vi "根据监测浓度升序排列.vi"(11 "标液浓度输入":dbl[][](array[numeric])) -> (3 "输出数组":dbl[][](array[numeric]))   [LabVIEW 2016]
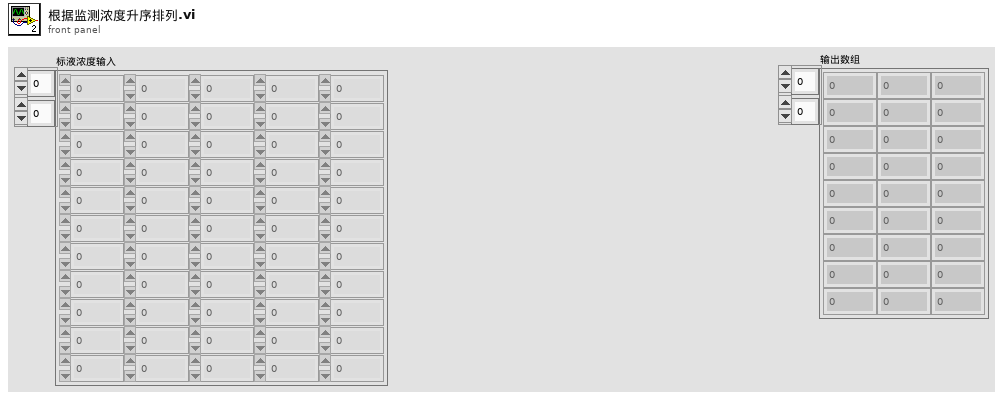
[diagram p1: front panel]
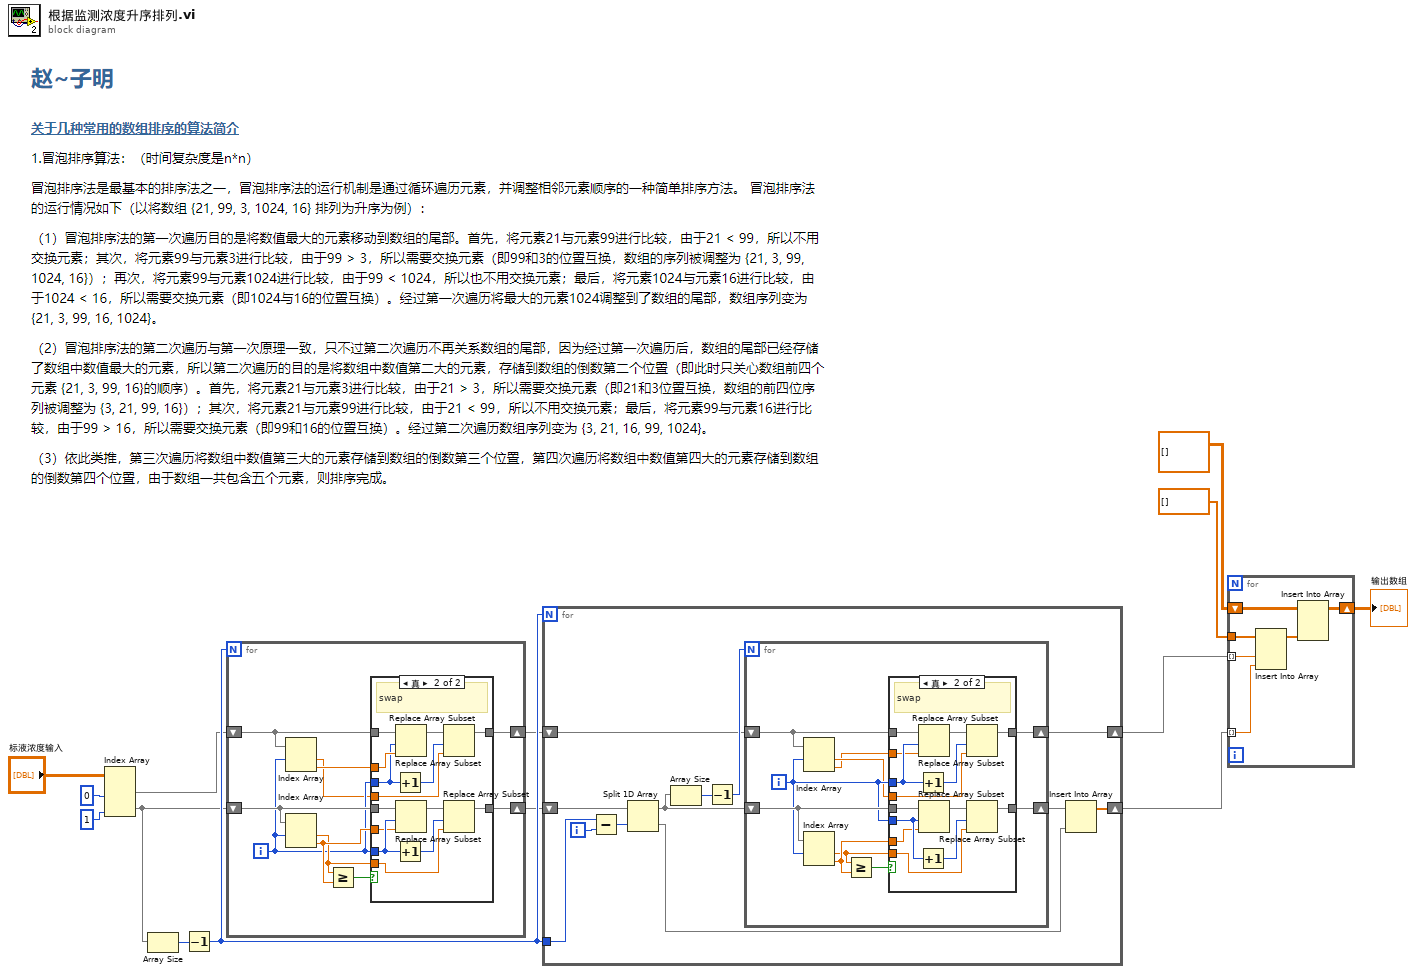
[diagram p0: block diagram]
diagram:
  n1 = Index Array(array="标液浓度输入", index (col) #1=0 ("禁用的索引 (列)"), index (col) #2=1 ("索引 (列)")) -> (element #1=w7:dbl[], element #2=w8:dbl[])  [unwired: 2 in]
  n2 = Array Size(array=w8) -> (size(s)=w11:i32)
  n3 = Decrement(x=w11) -> (x-1=w10:i32)
  n4 = for {
    N: w10 -> [_]
    shift-right: [w21] -> w9
    shift-left: w8 -> [w20]
    shift-right: [w17] -> w6
    shift-left: w7 -> [w19]
    i -> [w16]
    n5 = Index Array(array=w19, index #1=w16) -> (element #1=w15:dbl, element #2=w18:dbl)  [unwired: 1 in]
    n6 = Index Array(array=w20, index #1=w16) -> (element #1=w22:dbl, element #2=w23:dbl)  [unwired: 1 in]
    n7 = Greater Or Equal?(x=w22, y=w23) -> (x >= y?=w24:bool)
    n8 = case shown="真" w24 {
      tunnel: w20 -> [w26 w40]
      tunnel: w16 -> [_ w39]
      tunnel: w23 -> [_ w37]
      tunnel: w22 -> [_ w36]
      tunnel: [w26 w34] -> w21
      tunnel: w19 -> [w25 w30]
      tunnel: [w25 w33] -> w17
      tunnel: w18 -> [_ w29]
      tunnel: w16 -> [_ w28]
      tunnel: w15 -> [_ w27]
      frame False {
      }
      frame True {
        # "swap"
        n9 = Increment(x=w28) -> (x+1=w31:i32)
        n10 = Increment(x=w39) -> (x+1=w38:i32)
        n11 = Replace Array Subset(array=w30, new element=w29, index=w28) -> (w32:dbl[])
        n12 = Replace Array Subset(array=w40, new element=w37, index=w39) -> (w35:dbl[])
        n13 = Replace Array Subset(array=w32, new element=w27, index=w31) -> (w33:dbl[])
        n14 = Replace Array Subset(array=w35, new element=w36, index=w38) -> (w34:dbl[])
      }
    }
  }
  n15 = for {
    N: w10 -> [_]
    shift-right: [w45] -> w1
    shift-left: w9 -> [w50]
    tunnel: w10 -> [w48]
    shift-right: [w41] -> w2
    shift-left: w6 -> [w42]
    i -> [w44]
    n16 = Subtract(x=w48, y=w44) -> (x-y=w43:i32)
    n17 = Split 1D Array(array=w50, index=w43) -> (first subarray=w49:dbl[], second subarray=w46:dbl[])
    n18 = Array Size(array=w49) -> (size(s)=w52:i32)
    n19 = Decrement(x=w52) -> (x-1=w51:i32)
    n20 = for {
      N: w51 -> [_]
      shift-right: [w59] -> w47
      shift-left: w49 -> [w58]
      shift-right: [w57] -> w41
      shift-left: w42 -> [w55]
      i -> [w56]
      n21 = Index Array(array=w55, index #1=w56) -> (element #1=w54:dbl, element #2=w53:dbl)  [unwired: 1 in]
      n22 = Index Array(array=w58, index #1=w56) -> (element #1=w60:dbl, element #2=w61:dbl)  [unwired: 1 in]
      n23 = Greater Or Equal?(x=w60, y=w61) -> (x >= y?=w62:bool)
      n24 = case shown="真" w62 {
        tunnel: w58 -> [w64 w78]
        tunnel: w56 -> [_ w77]
        tunnel: w61 -> [_ w75]
        tunnel: w60 -> [_ w74]
        tunnel: [w64 w72] -> w59
        tunnel: w55 -> [w63 w69]
        tunnel: [w63 w68] -> w57
        tunnel: w56 -> [_ w67]
        tunnel: w54 -> [_ w66]
        tunnel: w53 -> [_ w65]
        frame False {
        }
        frame True {
          # "swap"
          n25 = Increment(x=w67) -> (x+1=w70:i32)
          n26 = Increment(x=w77) -> (x+1=w76:i32)
          n27 = Replace Array Subset(array=w69, new element=w65, index=w67) -> (w71:dbl[])
          n28 = Replace Array Subset(array=w78, new element=w75, index=w77) -> (w73:dbl[])
          n29 = Replace Array Subset(array=w71, new element=w66, index=w70) -> (w68:dbl[])
          n30 = Replace Array Subset(array=w73, new element=w74, index=w76) -> (w72:dbl[])
        }
      }
    }
    n31 = Insert Into Array(array=w47, new element=w46) -> (w45:dbl[])  [unwired: 1 in]
  }
  n32 = for {
    tunnel: w2 -> [w82] mode=indexing
    tunnel: w1 -> [w81] mode=indexing
    shift-right: [w80] -> w3
    shift-left: dbl[][] [] ("标液浓度") -> [w84]
    tunnel: dbl[] [] ("监测浓度") -> [w83]
    n33 = Insert Into Array(array=w83, new element #1=w82, new element #2=w81) -> (w79:dbl[])  [unwired: 1 in]
    n34 = Insert Into Array(array=w84, new element=w79) -> (w80:dbl[][])  [unwired: 2 in]
  }
  "输出数组" <- w3
